vi "svl_Init Arrays for Exp Avg (Resampled).vi"(0 "scaled signals":T1(array[cluster]) {"even angle signal" format="%.2f"; "dr" format="%.2f"; "r0" format="%.2f"}, 11 "error in (no error)":errorcluster) -> (4 "scaled signals":T1(array[cluster]) {"even angle signal" format="%.2f"; "dr" format="%.2f"; "r0" format="%.2f"}, 8 "initial values (impulse)":dbl[](array[numeric]) format="%.2f", 10 "dr":dbl, 14 "initial values (exp)":dbl[](array[numeric]) format="%.2f", 15 "error out":errorcluster)   [LabVIEW 2017]
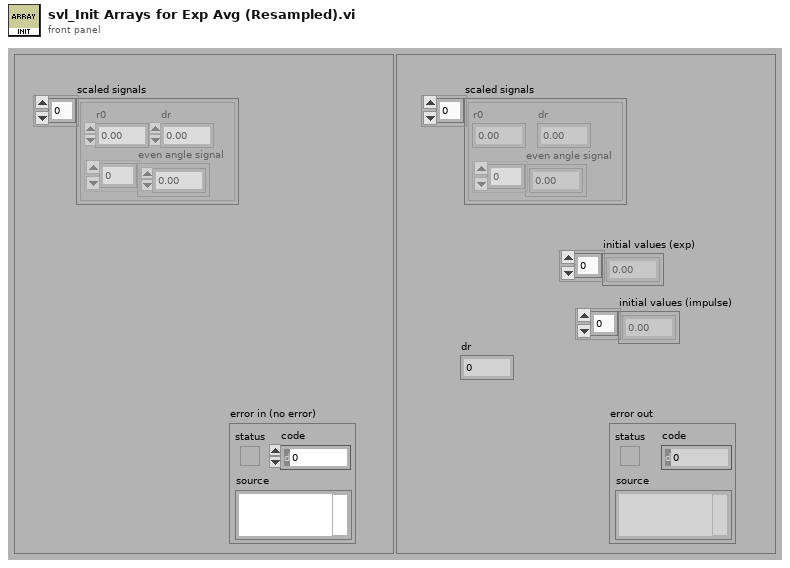
[diagram p1: front panel]
types:
  T1 = cluster{"r0":dbl, "dr":dbl, "even angle signal":dbl[]}[]
  T2 = cluster{"r0":dbl, "dr":dbl, "even angle signal":dbl[]}
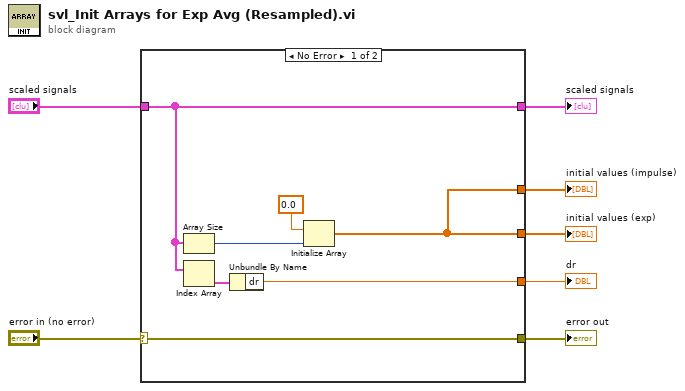
[diagram p0: block diagram]
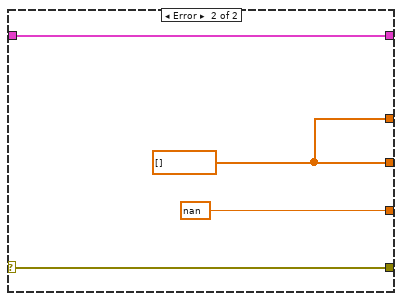
[diagram p2: hidden frame]
diagram:
  n1 = case shown="No Error" "error in (no error)" {
    selector: "error in (no error)" -> [w13 w17]
    tunnel: "scaled signals" -> [w11 w18]
    tunnel: [w10 w15] -> w7
    tunnel: [w11 w18] -> w4
    tunnel: [w13 w17] -> w3
    tunnel: [w10 w15] -> w2
    tunnel: [w8 nan ("dt")] -> w1
    frame No Error {
      n2 = Array Size(array=w11) -> (size(s)=w12:i32)
      n3 = Index Array(array=w11) -> (element=w9:T2)  [unwired: 1 in]
      n4 = Unbundle By Name(w9) -> ("dr"=w8:dbl)
      n5 = Initialize Array(0.0 ("squaredSum"), w12) -> (w10:dbl[])
    }
    frame Error {
      w15 = dbl[] []
    }
  }
  "initial values (exp)" <- w7
  "error out" <- w3
  "scaled signals" <- w4
  "initial values (impulse)" <- w2
  "dr" <- w1
